vi "WriteData.vi"(8 "error in (no error)":errorcluster, 11 "DAQ_Abstr in":refnum<class "DAQ_Abstr.lvclass">) -> (0 "error out":errorcluster, 3 "DAQ_Abstr out":refnum<class "DAQ_Abstr.lvclass">)   [LabVIEW 2025, in "DAQ_Abstr.lvlib" / "DAQ_Abstr.lvclass"]
uses:
  DAQ_Abstr.lvclass
  DAQ_Abstr.lvclass/DAQ_Abstr.ctl
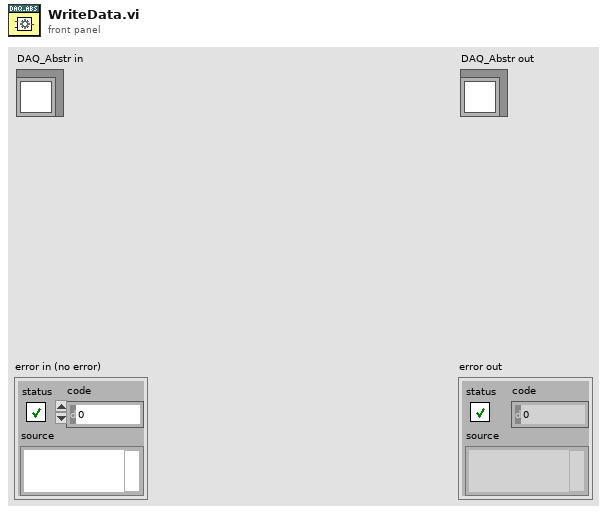
[diagram p1: front panel]
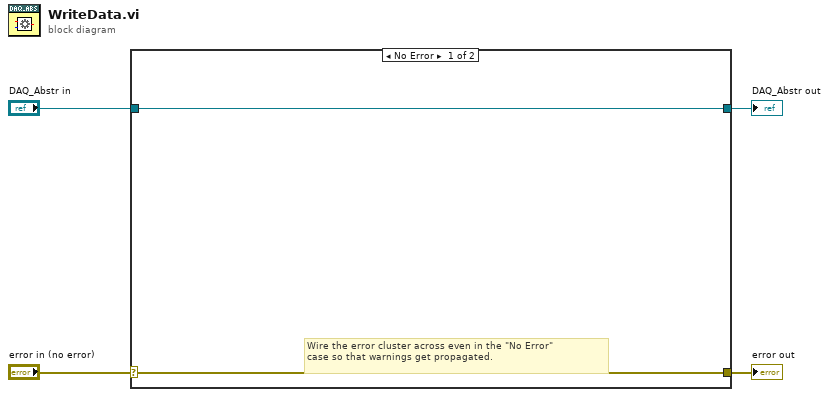
[diagram p0: block diagram]
diagram:
  n1 = case shown="No Error" "error in (no error)" {
    selector: "error in (no error)" -> [w5 w8]
    tunnel: [w5 w8] -> w3
    tunnel: [w6 w7] -> w1
    tunnel: "DAQ_Abstr in" -> [w6 w7]
    frame No Error {
      # "Wire the error cluster across even in the \"No Error\"\ncase so that warnings get propagated."
    }
    frame Error {
    }
  }
  "error out" <- w3
  "DAQ_Abstr out" <- w1
